vi "WallBallistics.vi"(2 "Gravitational Constant":dbl=386.09 format="%#_13g", 3 "Object Y Offset":dbl=96.0 format="%#_13g", 4 "Target Distance":dbl format="%#_13g") -> (0 "Angle (Radians)":dbl, 1 "Velocity":dbl)   [LabVIEW 2015]
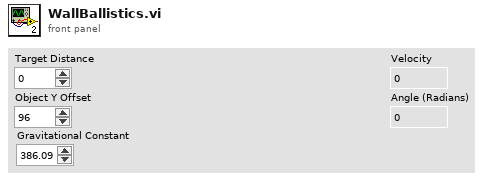
[diagram p1: front panel]
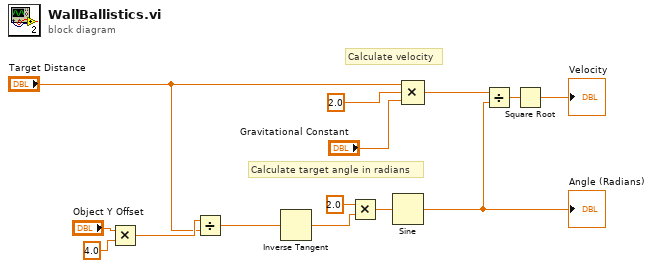
[diagram p0: block diagram]
diagram:
  # "Calculate target angle in radians"
  # "Calculate velocity"
  n1 = Multiply(x="Object Y Offset", y=4.0) -> (x*y=w5:dbl)
  n2 = Divide(x=w5, y="Target Distance") -> (x/y=w4:dbl)
  n3 = Inverse Tangent(1:w4) -> (0:w8:dbl)
  n4 = Multiply(x=2.0, y=w8) -> (x*y=w10:dbl)
  n5 = Sine(x=w10) -> (sin(x)=w3:dbl)
  "Angle (Radians)" <- w3
  n6 = Compound Arithmetic op=MULTIPLY("Target Distance", 2.0 ("y"), "Gravitational Constant") -> (w11:dbl)
  n7 = Divide(x=w11, y=w3) -> (x/y=w12:dbl)
  n8 = Square Root(x=w12) -> (sqrt(x)=→"Velocity":dbl)
